vi "ITX Folder to HDF5.vi"(8 "error in (no error)":errorcluster) -> (0 "error out":errorcluster)   [LabVIEW 2020]
panel:
  in  "Folder Path":path
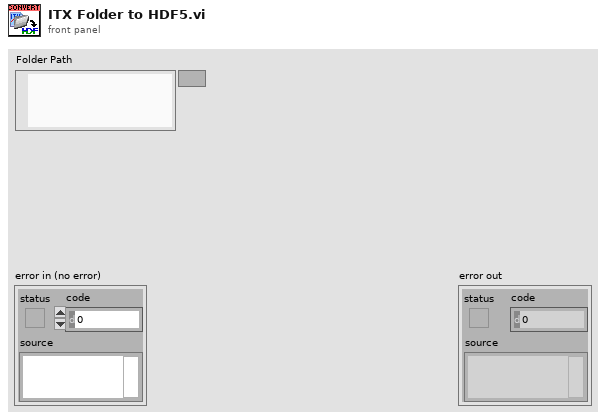
[diagram p1: front panel]
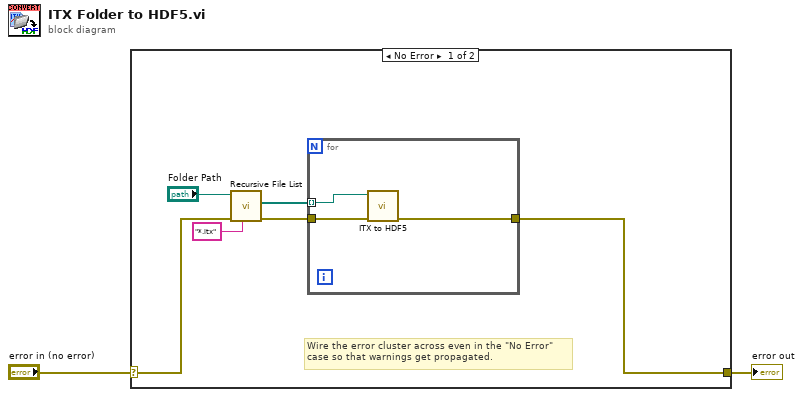
[diagram p0: block diagram]
diagram:
  n1 = case shown="No Error" "error in (no error)" {
    selector: "error in (no error)" -> [w4 w12]
    tunnel: [w3 w12] -> w1
    frame No Error {
      # "Wire the error cluster across even in the \"No Error\"\ncase so that warnings get propagated."
      n2 = call <vilib>:"Recursive File List.vi"("pattern"="*.itx", "error in (no error)"=w4, "Folder Path"="Folder Path") -> ("error out"=w5:errorcluster, "All Files in Dir"=w6:path[])  [unwired: 4 in, 3 out]
      n3 = for {
        tunnel: w6 -> [w9] mode=indexing
        tunnel: w5 -> [w11]
        tunnel: [w10] -> w3
        n4 = call "ITX to HDF5.vi"("error in (no error)"=w11, "file (use dialog)"=w9) -> ("error out"=w10:errorcluster)  [unwired: 9 in]
      }
    }
    frame Error {
    }
  }
  "error out" <- w1
